vi "updateAlly.vi"(8 "error in (no error)":errorcluster, 10 "Old Ally":refnum<class "Ally.lvclass">, 11 "New Ally from Vision":refnum<class "Ally.lvclass">) -> (0 "error out":errorcluster, 3 "Ally out":refnum<class "Ally.lvclass">)   [LabVIEW 2023, in "Ally.lvclass"]
uses:
  Ally.lvclass
  Utilities_class/Utilities.lvclass
  Robot_class/Robot.lvclass
  Team_class/Team.lvclass/Team.ctl
  Robot_class/Robot.lvclass/Robot.ctl
  Object_class/Object.lvclass/Object.ctl
  Object_class/Read x.vi
  Object_class/Read y.vi
  Robot_class/Read orientation.vi
  Robot_class/Read est_v_norm.vi
  Robot_class/Read est_v_tang.vi
  Object_class/Read pos_est_x.vi
  Object_class/Read pos_est_y.vi
  Robot_class/Read role.vi
  Object_class/Write x.vi
  Object_class/Write y.vi
  Robot_class/Write orientation.vi
  Robot_class/Write est_v_norm.vi
  Robot_class/Write est_v_tang.vi
  Object_class/Write pos_est_x.vi
  Object_class/Write pos_est_y.vi
  Robot_class/Write role.vi
  Robot_class/Read id.vi
  Team_class/Read RobotRef.vi
  Team_class/Write RobotRef.vi
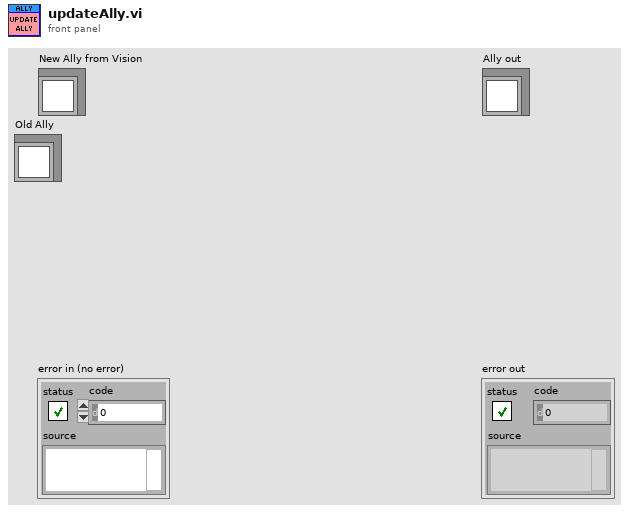
[diagram p1: front panel]
types:
  T1 = typedef "roles.ctl" = enum16{"BallChallengerAttackerVSS", "NormalAttackerVSS", "AttackerAimGoalVSS", "DefenderAreaVSS", "KeeperVSS", "Tabler", "TableFinalizer", "PrepareRollToPassRoller", "PrepareRollToPassReceiver", "SimplePassRoll", "SimplePassRollReceiver", "PenaltyDefense", "PreparePassReceiver 2", "PreparePassReceiver 1", "PassObserver", "Timeout", "Goto", "ZigZag", "None", "BallOutOfField", "DefenderArea", "Duelist", "AttackerStop", "FollowAttacker", "KeeperRole", "KickPenalty", "AttackerAimGoal", "AttackerBlock", "Marker", "Halt", "Shoot", "PassKicker", "PassReceiver", "TestRole", "PenaltyAttacker"}
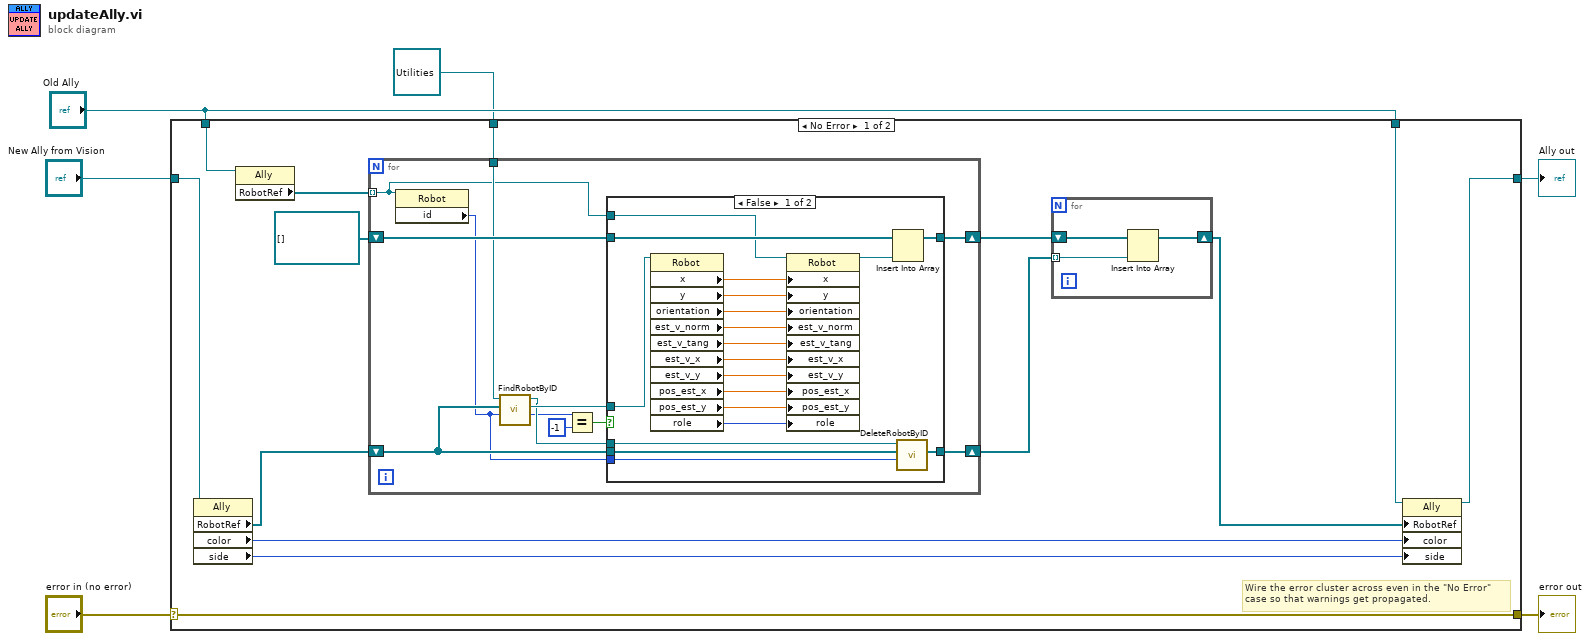
[diagram p0: block diagram]
diagram:
  n1 = case shown="No Error" "error in (no error)" {
    selector: "error in (no error)" -> [w20 w58]
    tunnel: [w20 w58] -> w5
    tunnel: [w18 w57] -> w3
    tunnel: "New Ally from Vision" -> [w19 w57]
    tunnel: "Old Ally" -> [w17 _]
    tunnel: "Old Ally" -> [w14 _]
    tunnel: refnum<class "Utilities.lvclass"> refnum ("Utilities in") -> [w10 _]
    frame No Error {
      # "Wire the error cluster across even in the \"No Error\"\ncase so that warnings get propagated."
      n2 = property class="Ally"(reference=w19) -> ("RobotRef"=w13:refnum<class "Robot.lvclass">[], "color"=w16:enum16{"Azul", "Amarelo"}, "side"=w15:enum16{"Esquerdo", "Direito"})  [unwired: 1 in, 2 out]
      n3 = property class="Ally"(reference=w14) -> ("RobotRef"=w12:refnum<class "Robot.lvclass">[])  [unwired: 1 in, 2 out]
      n4 = for {
        tunnel: w12 -> [w24] mode=indexing
        shift-right: [w34] -> w9
        shift-left: refnum<class "Robot.lvclass">[] [] -> [w33]
        tunnel: w10 -> [w32]
        shift-right: [w29] -> w8
        shift-left: w13 -> [w31]
        n5 = property class="Robot"(reference=w24) -> ("id"=w30:i32)  [unwired: 1 in, 2 out]
        n6 = call-dynamic "FindRobotByID.vi"("id"=w30, "RobotRef"=w31, "Utilities in"=w32) -> ("index"=w26:i32, "Robot"=w35:refnum<class "Robot.lvclass">, "Utilities out"=w28:refnum<class "Utilities.lvclass">)  [unwired: 5 in, 1 out]
        n7 = Equal?(x=w26, y=-1) -> (x = y?=w27:bool)
        n8 = case shown="False" w27 {
          tunnel: w35 -> [w46 _]
          tunnel: [w54 w56] -> w34
          tunnel: w33 -> [w53 w56]
          tunnel: w31 -> [w52 w55]
          tunnel: w30 -> [w51 _]
          tunnel: [w50 w55] -> w29
          tunnel: w28 -> [w49 _]
          tunnel: w24 -> [w48 _]
          frame False {
            n9 = property class="Robot"(reference=w46) -> ("x"=w45:dbl, "y"=w44:dbl, "orientation"=w43:dbl, "est_v_norm"=w42:dbl, "est_v_tang"=w41:dbl, "est_v_x"=w40:dbl, "est_v_y"=w39:dbl, "pos_est_x"=w38:dbl, "pos_est_y"=w37:dbl, "role"=w36:T1)  [unwired: 1 in, 2 out]
            n10 = property class="Robot"(reference=w48, "x"=w45, "y"=w44, "orientation"=w43, "est_v_norm"=w42, "est_v_tang"=w41, "est_v_x"=w40, "est_v_y"=w39, "pos_est_x"=w38, "pos_est_y"=w37, "role"=w36) -> (reference out=w47:refnum<class "Robot.lvclass">)  [unwired: 1 in, 1 out]
            n11 = Insert Into Array(array=w53, new element=w47) -> (w54:refnum<class "Robot.lvclass">[])  [unwired: 1 in]
            n12 = call-dynamic "DeleteRobotByID.vi"("id"=w51, "RobotRef"=w52, "Utilities in"=w49) -> ("RobotRef out"=w50:refnum<class "Robot.lvclass">[])  [unwired: 6 in, 2 out]
          }
          frame True {
          }
        }
      }
      n13 = for {
        shift-right: [w21] -> w7
        shift-left: w9 -> [w23]
        tunnel: w8 -> [w22] mode=indexing
        n14 = Insert Into Array(array=w23, new element=w22) -> (w21:refnum<class "Robot.lvclass">[])  [unwired: 1 in]
      }
      n15 = property class="Ally"(reference=w17, "RobotRef"=w7, "color"=w16, "side"=w15) -> (reference out=w18:refnum<class "Ally.lvclass">)  [unwired: 1 in, 1 out]
    }
    frame Error {
    }
  }
  "error out" <- w5
  "Ally out" <- w3
